vi "GetAlazar_SaveToFile_25_AVG - ATS-SDK.vi"(1 "File Array":string[](array[string]), 2 "lines per plane":i32, 5 "Digitizer Settings":T4={"Digitizer delay (us) "=0.0, "rf points per line"=2048, "lines per plane"=128, "Samp Rate (Hz)"=100000000.0, "Additional dig delay (us)"=0.0, "Voltage Scale"=0.4, "Pre-Looks"=0, "Offset delay (us)"=0.0, "bits A/D"=8, "Avg Num"=1, "DigTimeOut"=5.0, "Rel Dig Delay"=0.0, "Dig Ch"=0, "LeCroyCluster"={"LeCroy Channels"=[TRUE, FALSE, FALSE, FALSE], "LC read pt offset"=0.0, "Sweep Avg"=FALSE}, "Main Digitizer"=enum."NI Digitizer", "Dig Config"=enum."Single channel", "Digitizer ID Cluster"={"Acqiris/Alazar/SP ID"=[], "NI Instr Handles"=[], "LeCroy VISA"="", "GaGe Handle"={"Handle"=0, "Sample size"=0, "Resolution"=0, "Offset"=0, "Channels"=0, "Boards"=0}, "ATS Ref"="ATS9350", "Acqiris Address"=["PCI::INSTR0"], "ADQRef"=refnum, "adq_cu_ptr"=refnum}, "Trigger Settings"={"Trig Source"=1, "Trig Coupling"=0, "Trig Slope"=0, "Level (mV)"=1500.0}, "Bulk Acq"=FALSE, "Bulk Start Indexes"=[], "Data Ref RF"=refnum, "NI ID/Channel"=[], "Total Dig CH"=1, "Xtra Ann Trig delay (us)"=10.0, "Fix Z Delay?"=FALSE, "One Way Transmission?"=FALSE, "Data Ref Log"=refnum} {"Trigger Settings"."Trig Slope" items=["Positive", "Negative"]; "Trigger Settings"."Level (mV)" format="%.2f"; "Trigger Settings"."Trig Coupling" items=["DC 1 MOhm", "AC 1 MOhm", "DC 50 Ohm", "AC 50 Ohm"]; "Trigger Settings"."Trig Source" items=["Chan 1", "External"]; "Rel Dig Delay" format="%.2f"; "DigTimeOut" format="%.2f"; "Avg Num" min=1; "Offset delay (us)" format="%.2f"; "Additional dig delay (us)" format="%.2f"; "Digitizer delay (us)" format="%.2f"}, 7 "AlazarCluster":T8, 9 "Ann Array Params":T1={"Synth Foc?"=FALSE, "Focal Zones"=41, "Switch T/R"=0, "Trans Geometry (mm)"={"Transducer"=0, "Geo Focus"=12.0, "a (radius)"=3.0, "# of rings"=5, "kerf space "=0.1, "Center Freq"=12.0}, "Sub Ap Excite?"=FALSE, "Full Array Scan?"=FALSE, "Xmt/Rcv"={"XMIT"=[TRUE, TRUE, TRUE, TRUE, TRUE], "RCV"=[TRUE, TRUE, TRUE, TRUE, TRUE]}, "PulseSpacing (us)"=0.0, "Xmit Ring"=0, "XMIT CHS"=0, "RCV CHS"=0, "GPU?"=FALSE, "Save TIFF?"=FALSE, "downfactor"=1, "RCV 1CH"=0} {"RCV 1CH" items=["All", "1", "2", "3", "4", "5"]; "Trans Geometry (mm)"."Transducer" items=["6D 12R 40 MHz"=0, "10D 31R 20 MHz"=1, "10D 23R 20 MHz"=2, "6D 23R 40 MHz"=3, "4.5D 10.7R 40 MHz"=4, "9D 23.5R 20 MHz"=5, "9D 25.8R 20MHz"=6, "Enter"=99]; "Switch T/R" min=1 max=5 step=1}, 11 "errorin":errorcluster) -> (3 "Gain Array":T9(array[cluster]), 6 "VGain (dB)":dbl, 8 "data out":i16[][][](array[numeric]), 14 "Raw VGain (scale)":dbl, 15 "error out":errorcluster)   [LabVIEW 2022 SP3]
uses:
  -DigitizerRoutines/DigitizerSettings.ctl
  -DigitizerRoutines/Digitizer.ctl
  -DigitizerRoutines/DigConfig.ctl
  -DigitizerRoutines/DigitizerID.ctl
  C:/Windows/System32/ADQAPI_dotNet_helper.dll
  Annular Array/-AnnularRoutines/AnnularArray.ctl
  Annular Array/-AnnularRoutines/TransGeometry.ctl
  Annular Array/-AnnularRoutines/ArrayGeometry.ctl
panel:
  out "read time":u32
  out "save time":u32
  out "Numeric":i32
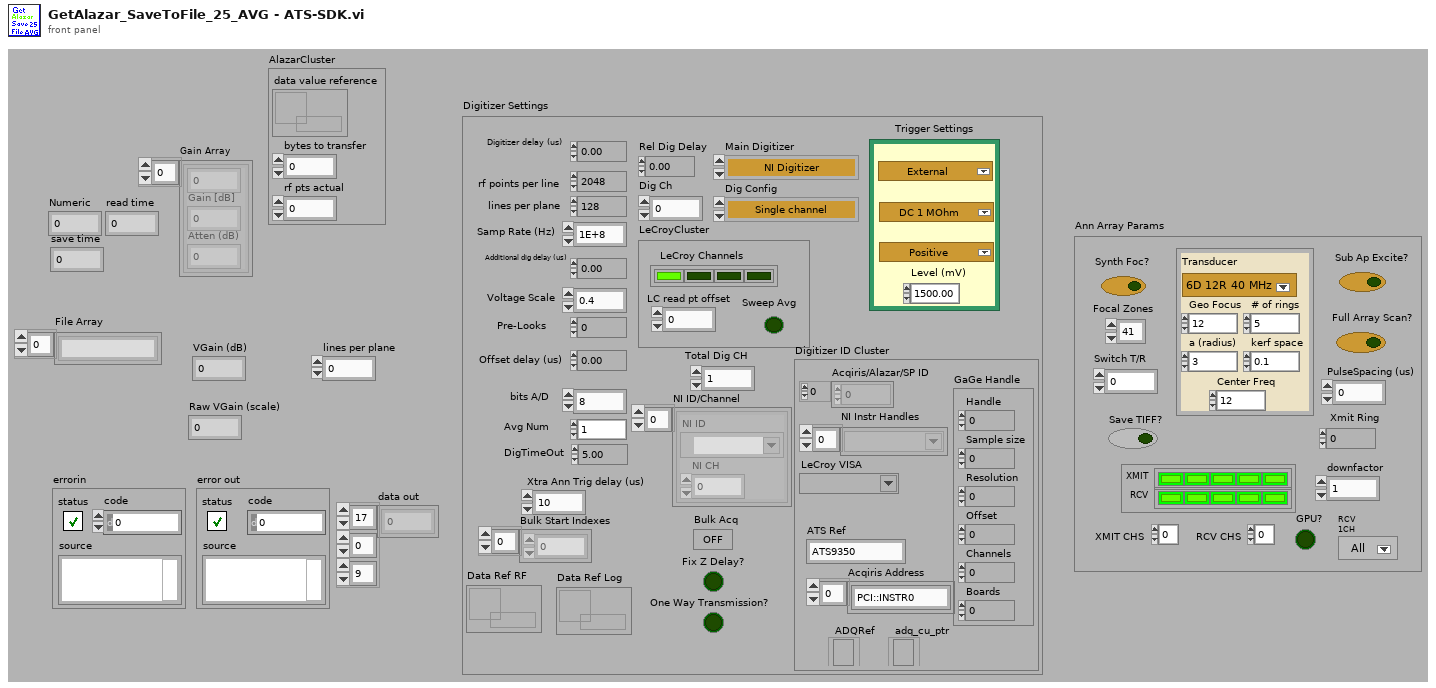
[diagram p1: front panel]
types:
  T1 = typedef "AnnularArray.ctl" = cluster{"Synth Foc?":bool, "Focal Zones":i16, "Switch T/R":i16, "Trans Geometry (mm)":T2, "Sub Ap Excite?":bool, "Full Array Scan?":bool, "Xmt/Rcv":cluster{"XMIT":bool[], "RCV":bool[]}, "PulseSpacing (us)":sgl, "Xmit Ring":i32, "XMIT CHS":u8, "RCV CHS":u8, "GPU?":bool, "Save TIFF?":bool, "downfactor":i32, "RCV 1CH":u16}
  T2 = typedef "TransGeometry.ctl" = cluster{"Transducer":T3, "Geo Focus":dbl, "a (radius)":dbl, "# of rings":i32, "kerf space ":dbl, "Center Freq":dbl}
  T3 = typedef "ArrayGeometry.ctl" = u16
  T4 = typedef "DigitizerSettings.ctl" = cluster{"Digitizer delay (us) ":dbl, "rf points per line":i32, "lines per plane":i32, "Samp Rate (Hz)":dbl, "Additional dig delay (us)":dbl, "Voltage Scale":dbl, "Pre-Looks":i32, "Offset delay (us)":dbl, "bits A/D":i8, "Avg Num":i32, "DigTimeOut":sgl, "Rel Dig Delay":sgl, "Dig Ch":i32, "LeCroyCluster":cluster{"LeCroy Channels":bool[], "LC read pt offset":dbl, "Sweep Avg":bool}, "Main Digitizer":T5, "Dig Config":T6, "Digitizer ID Cluster":T7, "Trigger Settings":cluster{"Trig Source":u16, "Trig Coupling":u16, "Trig Slope":u16, "Level (mV)":dbl}, "Bulk Acq":bool, "Bulk Start Indexes":i32[], "Data Ref RF":refnum<data-value>, "NI ID/Channel":cluster{"NI ID":refnum<k15>, "NI CH":i32}[], "Total Dig CH":i32, "Xtra Ann Trig delay (us)":dbl, "Fix Z Delay?":bool, "One Way Transmission?":bool, "Data Ref Log":refnum<data-value>}
  T5 = typedef "Digitizer.ctl" = enum16{"Acqiris Digitizer", "NI Digitizer", "LeCroy", "GaGe", "AlazarTech", "No Digitizer", "Teledyne"}
  T6 = typedef "DigConfig.ctl" = enum16{"Single channel", "2 Chans w/ 2 Acqiris", "2 Chans w/ 1 Acqiris", "5-CH Pulser New", "5-CH pulser w/ ann array", "5-pass style ann array", "Empty"}
  T7 = typedef "DigitizerID.ctl" = cluster{"Acqiris/Alazar/SP ID":u32[], "NI Instr Handles":refnum<k15>[], "LeCroy VISA":refnum<visa-resource-name>, "GaGe Handle":cluster{"Handle":u32, "Sample size":u32, "Resolution":i32, "Offset":i32, "Channels":u32, "Boards":u32}, "ATS Ref":string, "Acqiris Address":string[], "ADQRef":refnum<k24>, "adq_cu_ptr":refnum<k24>}
  T8 = cluster{"data value reference":refnum<data-value>, "bytes to transfer":u32, "rf pts actual":u32}
  T9 = cluster{sgl, "Gain [dB]  ":sgl, "Atten (dB)":sgl}[]
  T10 = cluster{"wfm":i16[][], "max queue size (-1, unlimited)":i32}
  T11 = cluster{sgl, "Gain [dB]  ":sgl, "Atten (dB)":sgl}
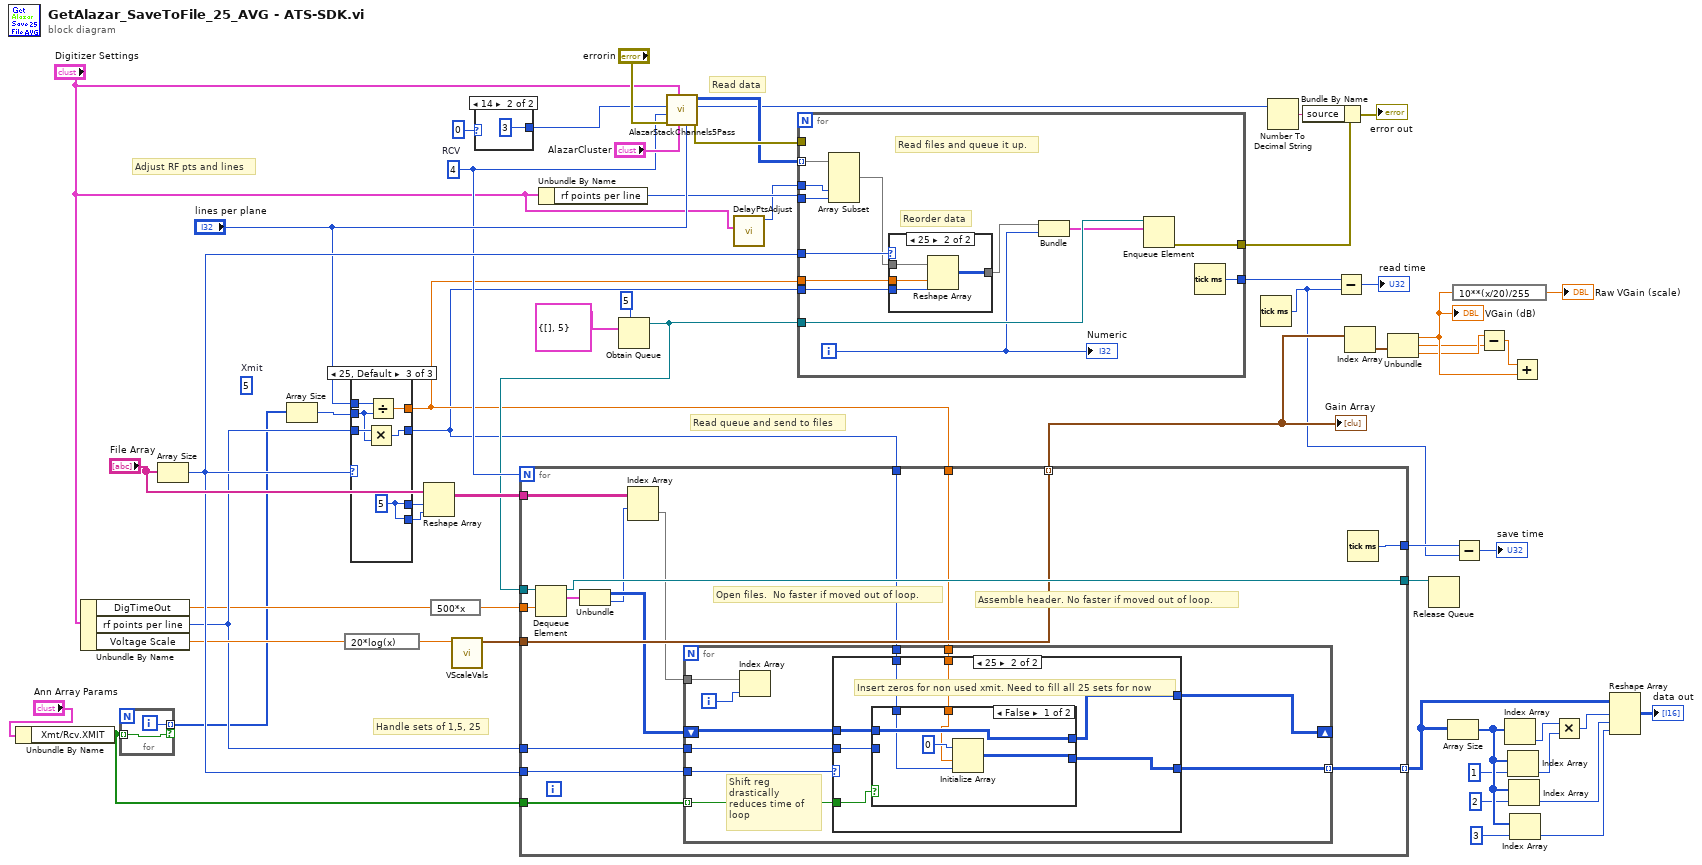
[diagram p0: block diagram]
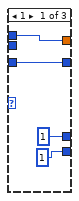
[diagram p4: hidden frame]
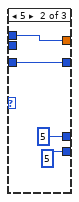
[diagram p5: hidden frame]
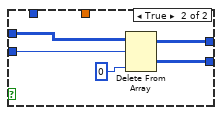
[diagram p7: hidden frame]
diagram:
  (unwired) 5  # Xmit
  w11 = 4  # RCV
  # "Read data"
  # "Adjust RF pts and lines"
  # "Handle sets of 1,5, 25"
  # "Read queue and send to files"
  n1 = Unbundle By Name("Ann Array Params") -> ("Xmt/Rcv.XMIT"=w4:bool[])
  n2 = Unbundle By Name("Digitizer Settings") -> ("DigTimeOut"=w14:sgl, "rf points per line"=w21:i32, "Voltage Scale"=w22:dbl)
  n3 = for {
    tunnel: w4 -> [w60] mode=indexing
    tunnel: [w61] -> w1 mode=indexing if=w60
    i -> [w61]
  }
  n4 = Array Size(array="File Array") -> (size(s)=w40:i32)
  n5 = Array Size(array=w1) -> (size(s)=w5:i32)
  n6 = expression code="20*log(x)"(w22) -> (w38:dbl)
  n7 = case shown="25, Default" w40 {
    tunnel: [1 5 w75] -> w43
    tunnel: [w64 w68 w71] -> w2
    tunnel: w21 -> [w64 w68 w72]
    tunnel: [w63 w67 w73] -> w3
    tunnel: "lines per plane" -> [w63 w67 w74]
    tunnel: [1 5 w75] -> w42
    tunnel: w5 -> [_ _ w70]
    frame 1 {
    }
    frame 5 {
    }
    frame 25, Default {
      w75 = 5
      n8 = Multiply(x=w72, y=w70) -> (x*y=w71:i32)
      n9 = Divide(x=w74, y=w70) -> (x/y=w73:dbl)
    }
  }
  n10 = Reshape Array("File Array", w43, w42) -> (w39:string[][])
  n11 = expression code="500*x"(w14) -> (w41:sgl)
  n12 = call "VScaleVals.vi"("Full Scale"=w38) -> ("Voltage Scale"=w37:T11)  [unwired: 8 in, 2 out]
  n13 = case shown="14" i8 0 ("bits A/D") {
    tunnel: [_ u16 3 ("Extra Shift")] -> w16
    frame 0, Default {
    }
    frame 14 {
    }
  }
  n14 = Unbundle By Name("Digitizer Settings") -> ("rf points per line"=w10:i32)
  n15 = Obtain Queue(max queue size (-1, unlimited)=5, element data type=T10 {"wfm"=[], "max queue size (-1, unlimited)"=5}) -> (queue out=w9:refnum<queue>)  [unwired: 3 in, 2 out]
  n16 = for {
    N: w11 -> [_]
    tunnel: w21 -> [w92]
    tunnel: [w84] -> w52 mode=indexing
    tunnel: w9 -> [w91]
    tunnel: [w89] -> w45
    tunnel: [w88] -> w49
    tunnel: w40 -> [w87]
    tunnel: w41 -> [w86]
    tunnel: w39 -> [w85]
    tunnel: w37 -> [w84]
    tunnel: [w81] -> w23 mode=indexing
    tunnel: w4 -> [w80]
    tunnel: w3 -> [w79]
    tunnel: w2 -> [w78]
    # "Open files.  No faster if moved out of loop."
    # "Assemble header. No faster if moved out of loop."
    n17 = Dequeue Element(queue=w91, timeout in ms (-1)=w86) -> (queue out=w89:refnum<queue>, element=w90:T10)  [unwired: 1 in, 2 out]
    n18 = Unbundle(w90) -> ("wfm"=w83:i16[][], "max queue size (-1, unlimited)"=w82:i32)
    n19 = Index Array(array=w85, index (row)=w82) -> (element=w77:string[])  [unwired: 1 in]
    n20 = for {
      tunnel: w92 -> [w102]
      tunnel: w87 -> [w100]
      shift-right: [w99] -> _
      shift-left: w83 -> [w101]
      tunnel: [w98] -> w81 mode=indexing
      tunnel: w80 -> [w97] mode=indexing
      tunnel: w79 -> [w96]
      tunnel: w78 -> [w95]
      tunnel: w77 -> [w94]
      i -> [w93]
      # "Shift reg drastically reduces time of loop"
      n21 = Index Array(array=w94, index=w93) -> ()  [unwired: 1 out]
      n22 = case shown="25" w100 {
        tunnel: w102 -> [_ w108]
        tunnel: w101 -> [w103 w110]
        tunnel: [w103 w109] -> w99
        tunnel: [w103 w107] -> w98
        tunnel: w97 -> [_ w106]
        tunnel: w96 -> [_ w105]
        tunnel: w95 -> [_ w104]
        frame 5, Default {
        }
        frame 25 {
          # "Insert zeros for non used xmit. Need to fill all 25 sets for now"
          n23 = case shown="False" w106 {
            tunnel: w110 -> [w113 w120]
            tunnel: [w113 w119] -> w109
            tunnel: w108 -> [_ w118]
            tunnel: [w114 w116] -> w107
            tunnel: w105 -> [w112 _]
            tunnel: w104 -> [w111 _]
            frame False {
              n24 = Initialize Array(i16 0, w112, w111) -> (w114:i16[][])
            }
            frame True {
              n25 = Delete From Array(array=w120, length=w118, index (col)=0 ("index (row)")) -> (deleted portion=w116:i16[][], array with subset deleted=w119:i16[][])  [unwired: 1 in]
            }
          }
        }
      }
    }
    n26 = Tick Count (ms)() -> (millisecond timer value=w88:u32)
  }
  "Gain Array" <- w52
  n27 = call "AlazarStackChannels5Pass.vi"("lines per plane"="lines per plane", "AlazarCluster"="AlazarCluster", "Digitizer Settings"="Digitizer Settings", "error in"="errorin", "Channels"=w11, "Extra Shift"=w16) -> ("error out"=w19:errorcluster, "Return Code"=w13:u32, "ChStackDataOut"=w15:i16[][][])  [unwired: 2 in, 1 out]
  n28 = call "DelayPtsAdjust.vi"("Digitizer Settings"="Digitizer Settings") -> ("PostDelayCorrection"=w7:u32)  [unwired: 9 in, 1 out]
  n29 = for {
    tunnel: w9 -> [w133]
    tunnel: [w131] -> w50
    tunnel: [w130] -> w36
    tunnel: w40 -> [w129]
    tunnel: w3 -> [w128]
    tunnel: w2 -> [w127]
    tunnel: w15 -> [w125] mode=indexing
    tunnel: w10 -> [w124]
    tunnel: w19 -> [_]
    tunnel: w7 -> [w121]
    i -> [w122]
    # "Read files and queue it up."
    # "Reorder data"
    n30 = Array Subset(array=w125, index (col)=w121, length (col)=w124) -> (w123:i16[][])  [unwired: 2 in]
    n31 = case shown="25" w129 {
      tunnel: w127 -> [_ w138]
      tunnel: w123 -> [w134 w137]
      tunnel: [w134 w136] -> w126
      tunnel: w128 -> [_ w135]
      frame 0, Default {
      }
      frame 25 {
        n32 = Reshape Array(w137, w135, w138) -> (w136:i16[][])
      }
    }
    n33 = Bundle(w126, w122) -> (w132:cluster{i16[][], i32})  [unwired: 1 in]
    n34 = Enqueue Element(queue=w133, element=w132) -> (error out=w130:errorcluster)  [unwired: 2 in, 2 out]
    n35 = Tick Count (ms)() -> (millisecond timer value=w131:u32)
    "Numeric" <- w122
  }
  n36 = Tick Count (ms)() -> (millisecond timer value=w48:u32)
  n37 = Number To Decimal String(number=w13) -> (decimal integer string=w35:string)  [unwired: 1 in]
  n38 = Bundle By Name(cluster=w36, "source"=w35) -> (→"error out":errorcluster)
  n39 = Subtract(x=w50, y=w48) -> (x-y=→"read time":u32)
  n40 = Index Array(array=w52) -> (element=w59:T11)  [unwired: 1 in]
  n41 = Unbundle(w59) -> (w58:sgl, "Gain [dB]"=w56:sgl, "Atten (dB)"=w57:sgl)
  "VGain (dB)" <- w58
  n42 = Release Queue(queue=w45) -> ()  [unwired: 2 in, 3 out]
  n43 = Array Size(array=w23) -> (size(s)=w33:i32[])
  n44 = expression code="10**(x/20)/255"(w58) -> (→"Raw VGain (scale)":sgl)
  n45 = Subtract(x=w49, y=w48) -> (x-y=→"save time":u32)
  n46 = Subtract(x=w57, y=w56) -> (x-y=w55:sgl)
  n47 = Index Array(array=w33) -> (element=w29:i32)  [unwired: 1 in]
  n48 = Index Array(array=w33, index=1) -> (element=w30:i32)
  n49 = Index Array(array=w33, index=2) -> (element=w32:i32)
  n50 = Index Array(array=w33, index=3) -> (element=w31:i32)
  n51 = Add(x=w55, y=w58) -> ()  [unwired: 1 out]
  n52 = Multiply(x=w29, y=w30) -> (x*y=w28:i32)
  n53 = Reshape Array(w23, w28, w32, w31) -> (→"data out":i16[][][])
